vi "clone.vi"(0 "reference":refnum<class "ChoiceNode.lvclass">, 5 "error in (no error)":errorcluster) -> (14 "reference out":refnum<class "ChoiceNode.lvclass">, 15 "clonedInterfaceNode":refnum<class "AbstractNode.lvclass">, 19 "error out":errorcluster)   [LabVIEW 2014, in "ChoiceNode.lvclass"]
doc: "public Object clone()"
uses:
  <resource>/Framework/Providers/Open_GDS/UML/ChoiceNode_class/ChoiceNode.lvclass
  <resource>/Framework/Providers/Open_GDS/UML/AbstractNode_class/AbstractNode.lvclass
  <resource>/Framework/Providers/Open_GDS/UML/MultiLineString_class/MultiLineString.lvclass
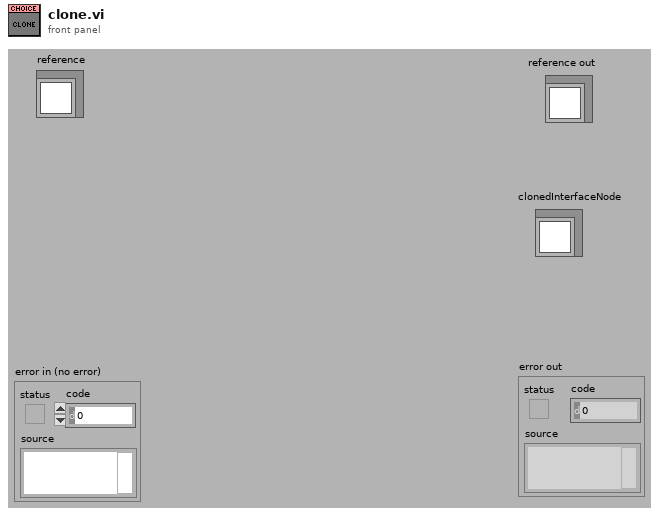
[diagram p1: front panel]
types:
  T1 = typedef "ChoiceNode.lvclass/ObjectAttributes.ctl" = cluster{"Base class":T2, "Text":refnum<class "MultiLineString.lvclass">, "DEFAULT_WIDTH":i32, "DEFAULT_HEIGHT":i32}
  T2 = typedef "RectangularNode.lvclass/ObjectAttributes.ctl" = cluster{"Base class":T3, "bounds":T4}
  T3 = typedef "AbstractNode.lvclass/ObjectAttributes.ctl" = cluster{"parent":refnum<class "AbstractNode.lvclass">, "children":refnum<class "AbstractNode.lvclass">[], "Hidden":bool}
  T4 = typedef "Rectangle Rectangle2D.ctl" = cluster{"x":dbl, "y":dbl, "width":dbl, "height":dbl}
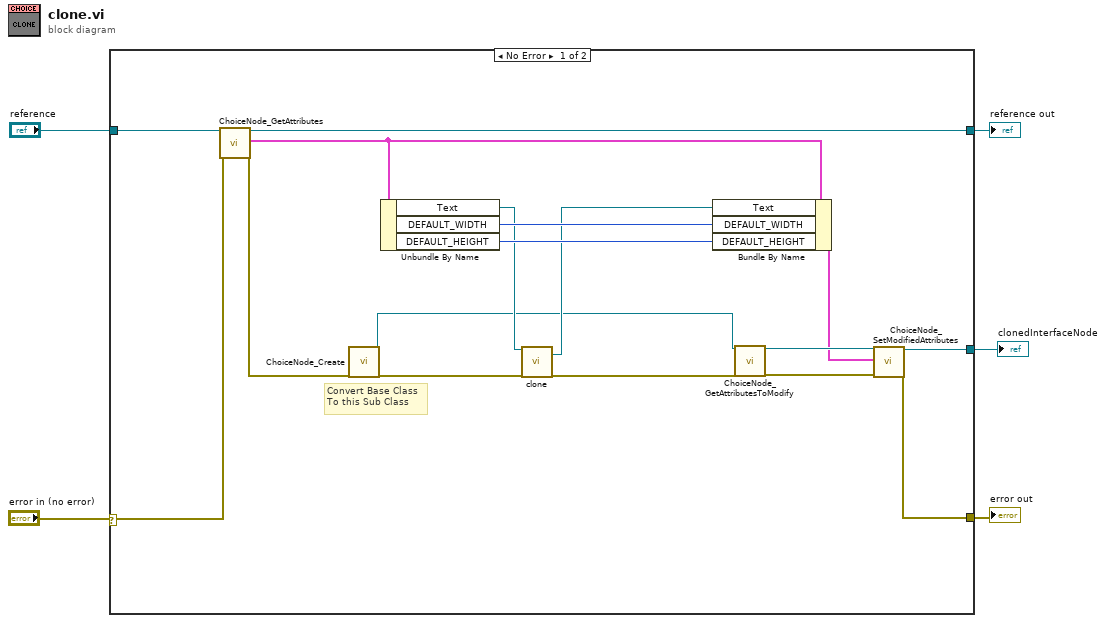
[diagram p0: block diagram]
diagram:
  n1 = case shown="No Error" "error in (no error)" {
    selector: "error in (no error)" -> [w20 w23]
    tunnel: "reference" -> [w22 w24]
    tunnel: [w21 w23] -> w4
    tunnel: [w7 w24] -> w3
    tunnel: [w19 _] -> w1
    frame No Error {
      # "Convert Base Class\nTo this Sub Class"
      n2 = call <resource>:"ChoiceNode_GetAttributes.vi"("reference in"=w22, "error in (no error)"=w20) -> ("reference out"=w7:refnum<class "ChoiceNode.lvclass">, "Attributes"=w8:T1, "error out"=w6:errorcluster)  [unwired: 15 out]
      n3 = call <resource>:"ChoiceNode_Create.vi"("error in (no error)"=w6) -> ("reference out"=w9:refnum<class "ChoiceNode.lvclass">, "error out"=w13:errorcluster)  [unwired: 16 in, 1 out]
      n4 = Unbundle By Name(w8) -> ("Text"=w12:refnum<class "MultiLineString.lvclass">, "DEFAULT_WIDTH"=w15:i32, "DEFAULT_HEIGHT"=w14:i32)
      n5 = call-dynamic "clone.vi"("reference"=w12, "error in (no error)"=w13) -> ("clonedMultiLineString"=w11:refnum<class "MultiLineString.lvclass">, "error out"=w10:errorcluster)  [unwired: 15 in, 1 out]
      n6 = Bundle By Name(cluster=w8, "Text"=w11, "DEFAULT_WIDTH"=w15, "DEFAULT_HEIGHT"=w14) -> (w16:T1)
      n7 = call <resource>:"ChoiceNode_GetAttributesToModify.vi"("reference in"=w9, "error in (no error)"=w10) -> ("reference out"=w18:refnum<class "ChoiceNode.lvclass">, "error out"=w17:errorcluster)  [unwired: 1 in, 15 out]
      n8 = call <resource>:"ChoiceNode_SetModifiedAttributes.vi"("reference in"=w18, "Attributes"=w16, "error in (no error)"=w17) -> ("reference out"=w19:refnum<class "ChoiceNode.lvclass">, "error out"=w21:errorcluster)  [unwired: 3 in, 12 out]
    }
    frame Error {
    }
  }
  "reference out" <- w3
  "error out" <- w4
  "clonedInterfaceNode" <- w1
